vi "LOAD -test.vi"(8 "error in (no error)":errorcluster, 9 "D(0)":dbl, 10 "Cp (1E-7 F)":dbl=1e-07, 11 "VISA resource name":refnum<visa-resource-name>) -> (0 "error out":errorcluster, 1 "X":dbl, 2 "R":dbl, 3 "VISA resource name out":refnum<visa-resource-name>)   [LabVIEW 2012]
panel:
  in  "Load Capacitance Threshold (1E-7 F)":dbl=1e-07
  in  "Load Supplementary Threshold (0)":dbl
  in  "Enable Load Correction (F: Disable) 2":bool
  in  "Load Correction  (0: Parallel - Dissipation Factor) 2":u16(ring) items=["Parallel - Dissipation Factor", "Parallel - Quality Factor", "Parallel - Conductance", "Parallel - Parallel Resistance", "Series - Dissipation Factor", "Series - Quality Factor", "Series- Series resistance"]
  in  "Load Correction  (0: Parallel - Dissipation Factor)":u16(ring) items=["Parallel - Dissipation Factor", "Parallel - Quality Factor", "Parallel - Conductance", "Parallel - Parallel Resistance", "Series - Dissipation Factor", "Series - Quality Factor", "Series- Series resistance"]
  in  "Enable Short Correction (F: Disable)":bool
  in  "Short Supplementary Threshold (0)":dbl
  in  "Short Capacitance Threshold (0)":dbl
  in  "Short Correction Type (0: Resistance- Reactance)":u16(ring) items=[" Resistance- Reactance", "Series Inductance- Series Resistance"]
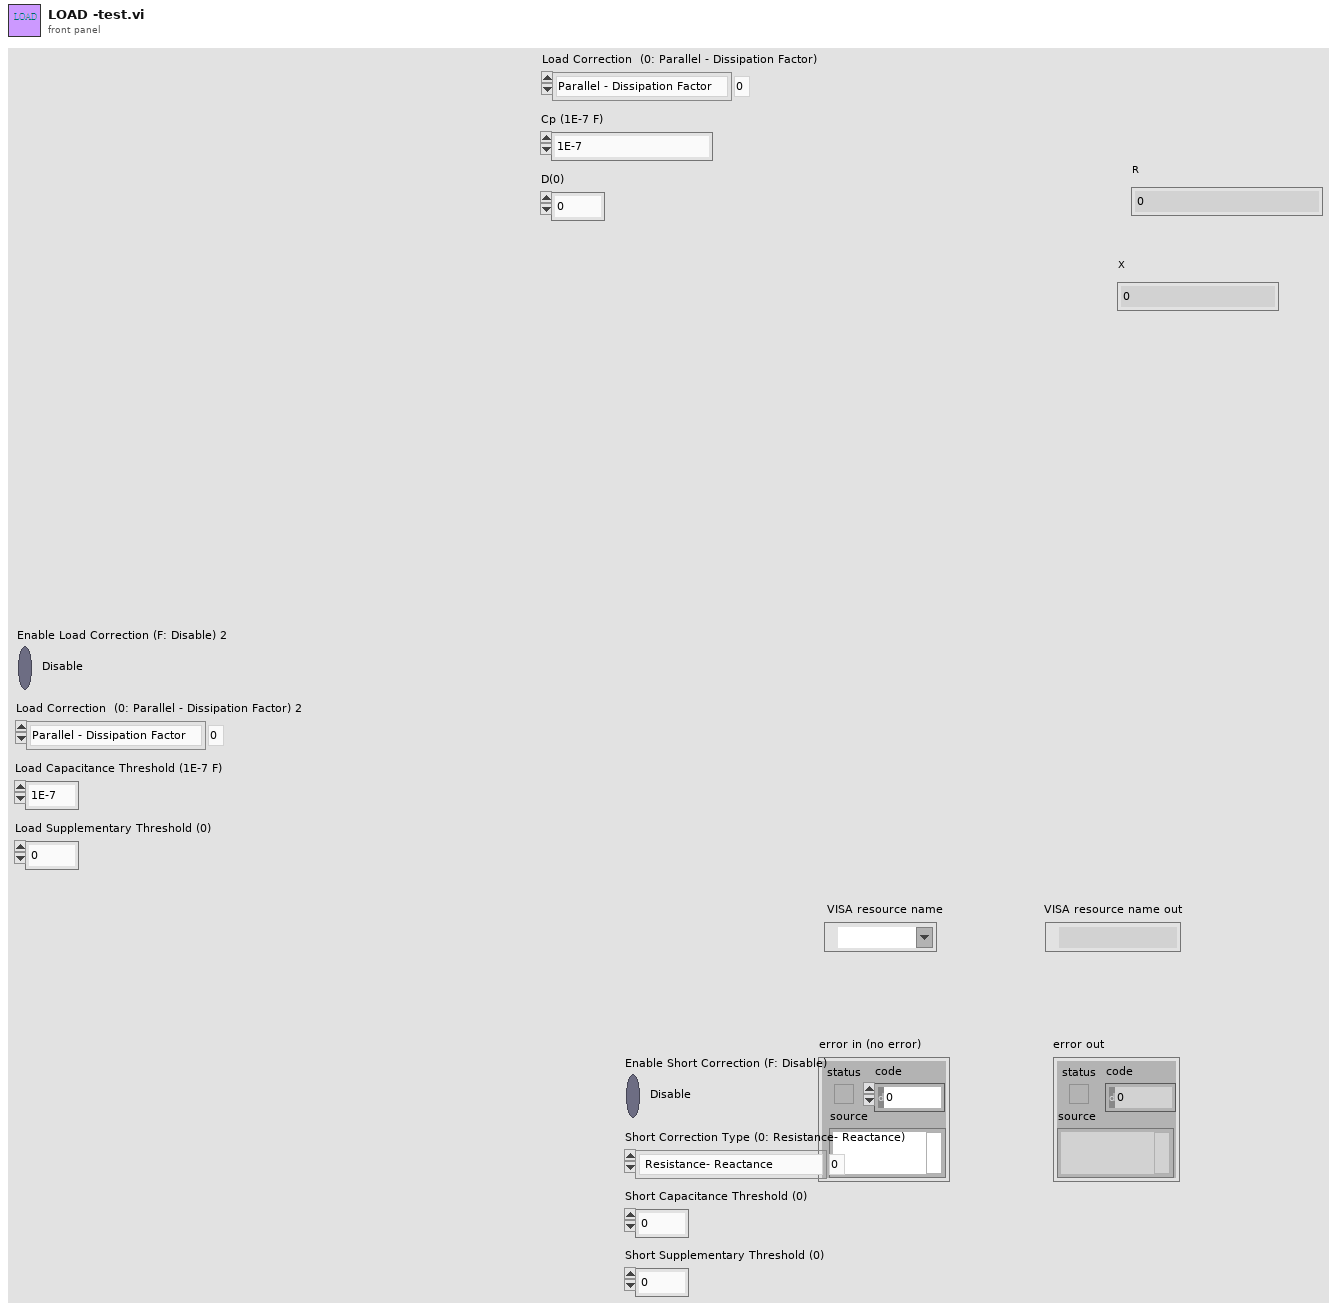
[diagram p1: front panel]
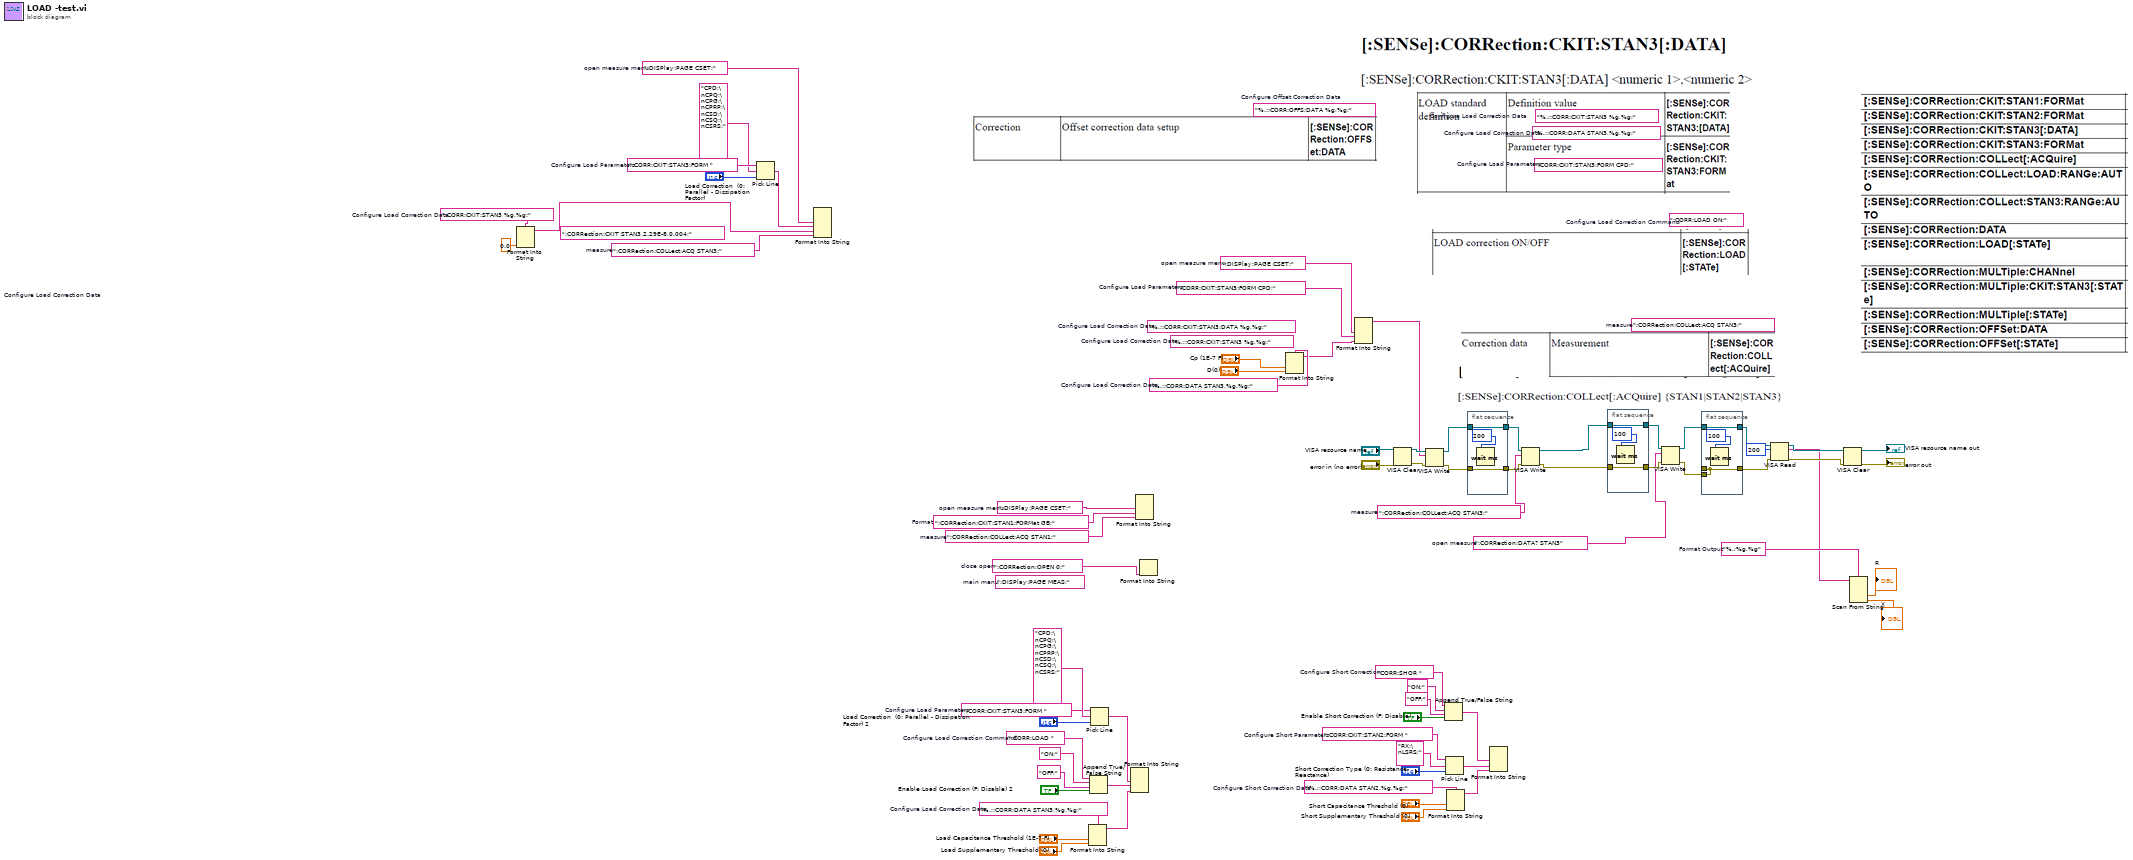
[diagram p0: block diagram]
diagram:
  w8 = "%.;%g,%g"  # Format Output
  w7 = ":CORRection:DATA? STAN3"  # open measure
  w18 = "%.;:CORR:DATA STAN3,%g,%g;"  # Configure Load Correction Data
  (unwired) "%.;:CORR:CKIT:STAN3:DATA %g,%g;"  # Configure Load Correction Data
  (unwired) "%.;:CORR:CKIT:STAN3 %g,%g;"  # Configure Load Correction Data
  (unwired) "%.;:CORR:DATA STAN3,%g,%g;"  # Configure Load Correction Data
  w19 = ":CORRection:COLLect:ACQ STAN3;"  # measure
  (unwired) "%.;:CORR:CKIT:STAN3 %g,%g;"  # Configure Load Correction Data
  (unwired) ":CORR:LOAD ON;"  # Configure Load Correction Command
  (unwired) ":CORRection:COLLect:ACQ STAN3;"  # measure
  (unwired) ":CORR:CKIT:STAN3:FORM CPD;"  # Configure Load Parameters
  (unwired) "%.;:CORR:OFFS:DATA %g,%g;"  # Configure Offset Correction Data
  w27 = 0.0 ("input 1")
  w29 = ":DISPlay:PAGE CSET;"  # open measure menu
  w28 = ":CORR:CKIT:STAN3:FORM CPD;"  # Configure Load Parameters
  w37 = "%.;:CORR:DATA STAN3,%g,%g;"  # Configure Load Correction Data
  w35 = ":CORR:CKIT:STAN3:FORM "  # Configure Load Parameters
  w31 = ":CORR:LOAD "  # Configure Load Correction Command
  w43 = ":CORR:CKIT:STAN3 %g,%g;"  # Configure Load Correction Data
  (unwired) ":CORRection:CKIT STAN3,2.29E-8,0.004;"  # Configure Load Correction Data
  w48 = ":CORRection:OPEN 0;"  # close open
  w49 = ":CORRection:COLLect:ACQ STAN1;"  # measure
  w50 = ":CORRection:CKIT:STAN1:FORMat GB;"  # Format
  (unwired) ":DISPlay:PAGE MEAS;"  # main menu
  w51 = ":DISPlay:PAGE CSET;"  # open measure menu
  w54 = ":CORR:CKIT:STAN3:FORM "  # Configure Load Parameters
  w45 = ":CORRection:COLLect:ACQ STAN3;"  # measure
  w60 = ":DISPlay:PAGE CSET;"  # open measure menu
  w65 = "%.;:CORR:DATA STAN2,%g,%g;"  # Configure Short Correction Data
  w69 = ":CORR:CKIT:STAN2:FORM "  # Configure Short Parameters
  w73 = "CORR:SHOR "  # Configure Short Correction
  n1 = Format Into String(format string=w43, w27, w27) -> (resulting string=w44:string)  [unwired: 2 in, 1 out]
  n2 = Pick Line(string ("")=w54, multi-line string="CPD;\nCPQ;\nCPG;\nCPRP;\nCSD;\nCSQ;\nCSRS;", line index="Load Correction  (0: Parallel - Dissipation Factor)") -> (output string=w52:string)
  n3 = Format Into String(w60, w52, w44, w45) -> ()  [unwired: 3 in, 2 out]
  n4 = Format Into String(format string=w37, "Load Capacitance Threshold (1E-7 F)", "Load Supplementary Threshold (0)") -> (resulting string=w41:string)  [unwired: 2 in, 1 out]
  n5 = Append True/False String(1:"Enable Load Correction (F: Disable) 2", 2:"OFF;" ("false string"), 3:"ON;" ("true string"), 4:w31) -> (0:w40:string)
  n6 = Pick Line(string ("")=w35, multi-line string="CPD;\nCPQ;\nCPG;\nCPRP;\nCSD;\nCSQ;\nCSRS;", line index="Load Correction  (0: Parallel - Dissipation Factor) 2") -> (output string=w42:string)
  n7 = Format Into String(w42, w40, w41) -> ()  [unwired: 3 in, 2 out]
  n8 = Format Into String(w51, w50, w49) -> ()  [unwired: 3 in, 2 out]
  n9 = Format Into String(w48) -> ()  [unwired: 3 in, 2 out]
  n10 = Format Into String(format string=w18, "Cp (1E-7 F)", "D(0)") -> (resulting string=w11:string)  [unwired: 2 in, 1 out]
  n11 = Format Into String(w29, w28, w11) -> (resulting string=w24:string)  [unwired: 3 in, 1 out]
  n12 = VISA Clear(VISA resource name="VISA resource name", error in (no error)="error in (no error)") -> (VISA resource name out=w59:refnum<visa-resource-name>, error out=w58:errorcluster)
  n13 = VISA Write(VISA resource name=w59, write buffer=w24, error in (no error)=w58) -> (VISA resource name out=w22:refnum<visa-resource-name>, error out=w21:errorcluster)  [unwired: 1 out]
  n14 = Append True/False String(1:"Enable Short Correction (F: Disable)", 2:"OFF;" ("true string"), 3:"ON;" ("true string"), 4:w73) -> (0:w62:string)
  n15 = Pick Line(string ("")=w69, multi-line string="RX;\nLSRS;", line index="Short Correction Type (0: Resistance- Reactance)") -> (output string=w63:string)
  n16 = Format Into String(format string=w65, "Short Capacitance Threshold (0)", "Short Supplementary Threshold (0)") -> (resulting string=w61:string)  [unwired: 2 in, 1 out]
  n17 = flat-sequence {
    tunnel: [w75] -> w23
    tunnel: w22 -> [w75]
    tunnel: w21 -> [w74]
    tunnel: [w74] -> w20
    frame #0 {
      n18 = Wait (ms)(milliseconds to wait=u32 200 ("byte count")) -> ()  [unwired: 1 out]
    }
  }
  n19 = Format Into String(w62, w63, w61) -> ()  [unwired: 3 in, 2 out]
  n20 = VISA Write(VISA resource name=w23, write buffer=w19, error in (no error)=w20) -> (VISA resource name out=w15:refnum<visa-resource-name>, error out=w14:errorcluster)  [unwired: 1 out]
  n21 = flat-sequence {
    tunnel: [w78] -> w16
    tunnel: w15 -> [w78]
    tunnel: w14 -> [w77]
    tunnel: [w77] -> w17
    frame #0 {
      n22 = Wait (ms)(milliseconds to wait=u32 100 ("byte count")) -> ()  [unwired: 1 out]
    }
  }
  n23 = VISA Write(VISA resource name=w16, write buffer=w7, error in (no error)=w17) -> (VISA resource name out=w13:refnum<visa-resource-name>, error out=w12:errorcluster)  [unwired: 1 out]
  n24 = flat-sequence {
    tunnel: [w81] -> w6
    tunnel: w13 -> [w81]
    tunnel: [w80] -> _
    tunnel: [w80] -> w5
    tunnel: w12 -> [w80]
    frame #0 {
      n25 = Wait (ms)(milliseconds to wait=u32 100 ("byte count")) -> ()  [unwired: 1 out]
    }
  }
  n26 = VISA Read(VISA resource name=w6, byte count=u32 200, error in (no error)=w5) -> (VISA resource name out=w4:refnum<visa-resource-name>, read buffer=w2:string, error out=w3:errorcluster)  [unwired: 1 out]
  n27 = VISA Clear(VISA resource name=w4, error in (no error)=w3) -> (VISA resource name out=→"VISA resource name out":refnum<visa-resource-name>, error out=→"error out":errorcluster)
  n28 = Scan From String(format string=w8, input string=w2) -> (output 1=→"R":dbl, output 2=→"X":dbl)  [unwired: 4 in, 3 out]
